vi "Init_Handler.vi"(8 "Error In":errorcluster caption="Entrée d'erreur", 11 "Donnees_Globales_IN":T1) -> (0 "Error Out":errorcluster, 3 "Donnees_Globale_Out":T1)   [LabVIEW 2019]
uses:
  Asc_State_Inputs.ctl
  Etat_Asc.ctl
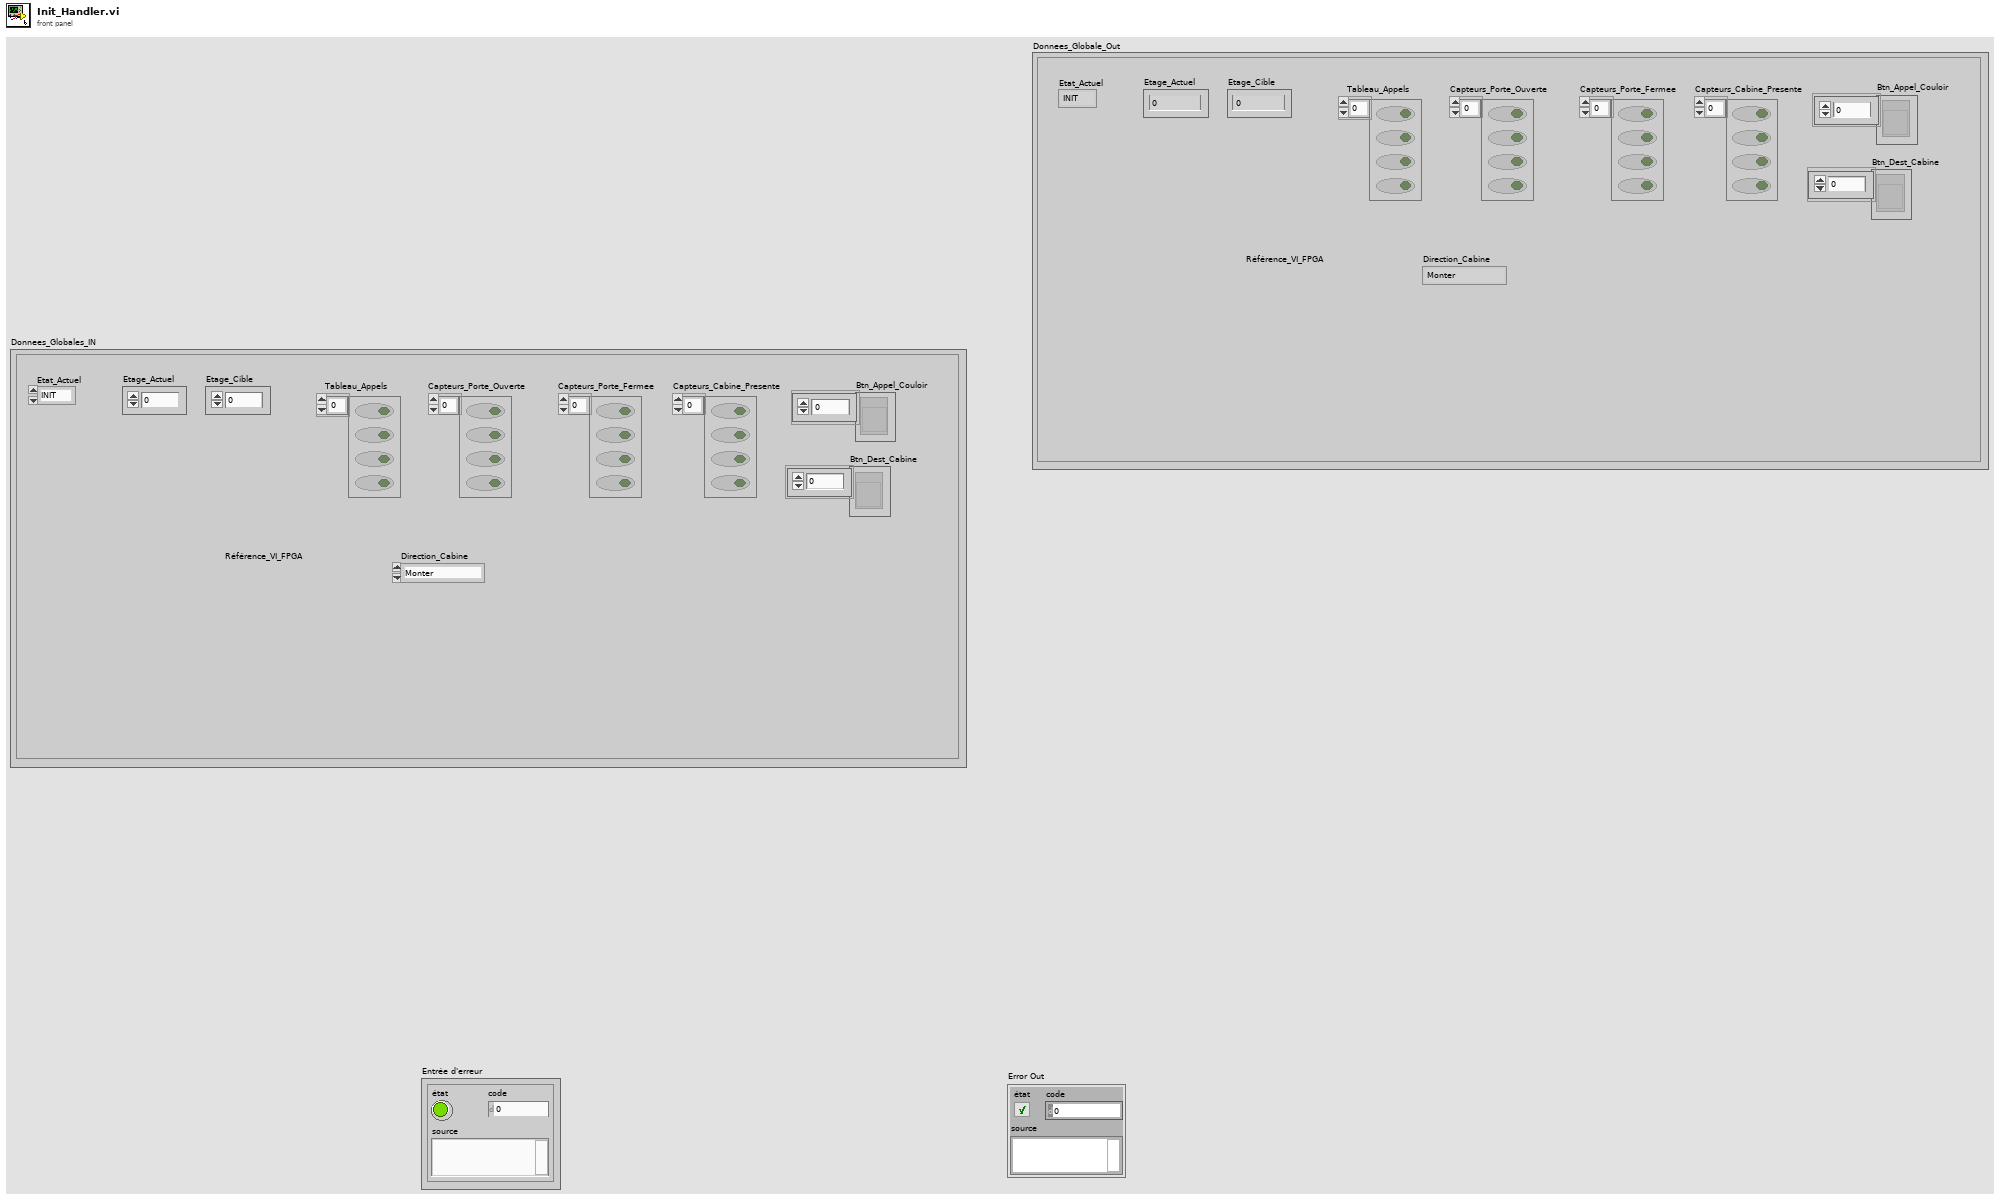
[diagram p1: front panel]
types:
  T1 = typedef "Asc_State_Inputs.ctl" = cluster{"Etage_Actuel":i32, "Etat_Actuel":T2, "Etage_Cible":i32, "Tableau_Appels":bool[], "Capteurs_Porte_Ouverte":bool[], "Capteurs_Porte_Fermee":bool[], "Capteurs_Cabine_Presente":bool[], "Btn_Appel_Couloir":refnum<vi>[], "Btn_Dest_Cabine":refnum<vi>[], "Référence_VI_FPGA":refnum<k20>, "Direction_Cabine":enum16{"Monter", "Descendre", "Arreter"}}
  T2 = typedef "Etat_Asc.ctl" = enum16{"INIT", "REPOS", "DEPLACEMENT", "OUVERTURE_PORTE", "ATTENTE_TEMPO", "FERMETURE_PORTE", "ARRET_URGENCE"}
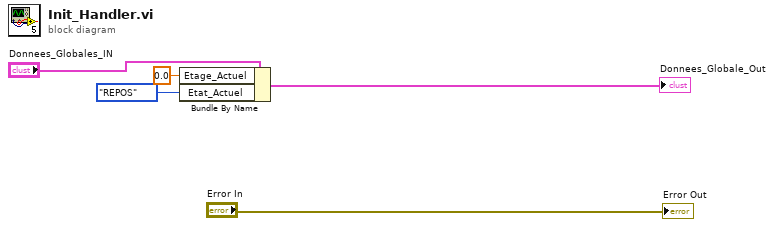
[diagram p0: block diagram]
diagram:
  n1 = Bundle By Name(cluster="Donnees_Globales_IN", "Etage_Actuel"=0.0, "Etat_Actuel"=Etat_Asc."REPOS") -> (→"Donnees_Globale_Out":T1)
  "Error Out" <- "Error In"
